vi "Start.vi"(7 "Plugin Name":string, 8 "error in (no error)":errorcluster, 10 "Index":i32, 11 "CIF_Plugin_UI in":refnum<class "CIF_UI.lvclass">) -> (0 "error out":errorcluster, 1 "Not Found":bool, 3 "CIF_Plugin_UI out":refnum<class "CIF_UI.lvclass">)   [LabVIEW 2021, in "CIF_UI.lvclass"]
uses:
  CIF_UI.lvclass
  CIF_UI.lvclass/CIF_UI.ctl
  CIFCore/Grpc/CIFCoreWrapper/CIFCoreWrapper.lvlib
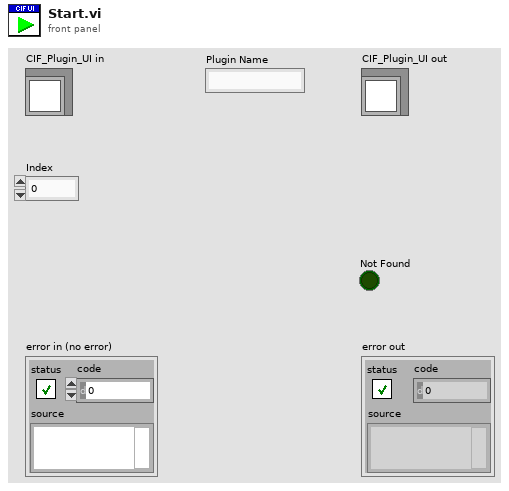
[diagram p1: front panel]
types:
  T1 = typedef "grpc-lvsupport-release.lvlib/grpcId.ctl" = u64
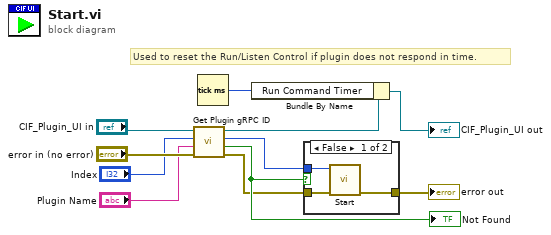
[diagram p0: block diagram]
diagram:
  # "Used to reset the Run/Listen Control if plugin does not respond in time."
  n1 = call "Get Plugin gRPC ID.vi"("error in (no error)"="error in (no error)", "Plugin Name"="Plugin Name", "Index"="Index", "CIF_UI in"="CIF_Plugin_UI in") -> ("error out"=w5:errorcluster, "Not Found"=w6:bool, "gRPC ID"=w7:T1, "CIF_UI out"=w3:refnum<class "CIF_UI.lvclass">)  [unwired: 3 in, 1 out]
  "Not Found" <- w6
  n2 = Tick Count (ms)() -> (millisecond timer value=w2:u32)
  n3 = Bundle By Name(cluster=w3, "Run Command Timer"=w2) -> (→"CIF_Plugin_UI out":refnum<class "CIF_UI.lvclass">)
  n4 = case shown="False" w6 {
    tunnel: w7 -> [w14 _]
    tunnel: w5 -> [w13 w15]
    tunnel: [w12 w15] -> w4
    frame False {
      n5 = call "Start.vi"("error in"=w13, "gRPC ID"=w14) -> ("error out"=w12:errorcluster)  [unwired: 8 in, 1 out]
    }
    frame True {
    }
  }
  "error out" <- w4
